vi "main.vi"() -> ()   [LabVIEW 2020]
uses:
  Monochromator/Monochromator.lvclass
  MonoStateFactory/MonoStateFactory.lvclass
  ts_labview_tcp/TCPServer/TCPServer.lvclass
  C:/Users/ecoughlin/repos/ss_monochromator_2/ts_labview_tcp/TCPCommunicator/TCPCommunicator.lvclass
  ts_labview_tcp/TCPComEvents/TCPComEvents.lvclass
  MonoCommunicator/MonoCommunicator.lvclass
  MonoPubSubData/MonoPubSubData.lvclass
  Typedefs/SWStatus.ctl
  ts_labview_tcp/TCPSettings/TCPSettings.lvclass
  MonoPubSubData/MonoPubSubData.lvclass/MonoPubSubData.ctl
  ts_labview_tcp/TCPComEvents/TCPComEvents.lvclass/TCPComEvents.ctl
  ts_labview_tcp/TCPCommunicator/TCPCommunicator.lvclass/TCPCommunicator.ctl
  MonoCommunicator/MonoCommunicator.lvclass/MonoCommunicator.ctl
  Monochromator/Monochromator.lvclass/Monochromator.ctl
  MonoSettings/Settings/ProcessSetting/ProcessSettings.lvclass
  C:/Users/ecoughlin/repos/ss_monochromator_2/WindowsController/MonoSettings/Settings/Settings/Setting.lvclass
  MonoSettings/Settings/Settings/Setting.lvclass/Setting.ctl
  ts_labview_tcp/TCPCommunicator/TCPCommunicator.lvclass
  MonoSettings/Settings/Settings/Setting.lvclass
  MonoSettings/Settings/ConfigurationFileReader/ConfigurationFileReader.lvclass
panel:
  out "TCP Connected":bool
  out "MonoID":string(combo)="Mono4"
  out "UniqueID":string="Mono1"
  # "Monochrmator"
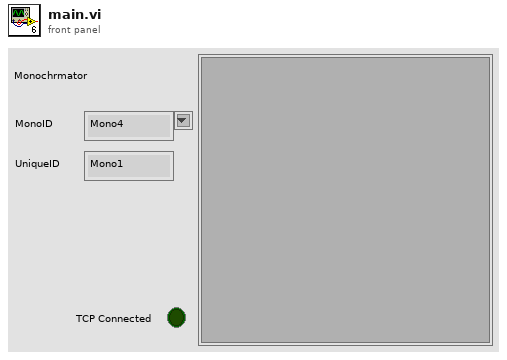
[diagram p1: front panel]
types:
  T1 = typedef "SWStatus.ctl" = enum16{"OfflineState", "ReadyState", "SettingUpState", "FaultState"}
  T2 = typedef "Settings.lvlib/ConfigurationTypedefs.lvlib/MonochromatorSettings.ctl" = cluster{"Force Init":bool, "WavelengthMin":T3, "WavelengthMax":T3, "SlitWidthMin":T4, "SlitWidthMax":T4, "timeout":dbl}
  T3 = typedef "wavelength.ctl" = dbl
  T4 = typedef "slitWidth.ctl" = dbl
  T5 = typedef "Settings.lvlib/ConfigurationTypedefs.lvlib/TCPConfiguration.ctl" = cluster{"IP":string, "port_low":u16, "port_up":u16, "connection_timeout ":i32, "reading_timeout":i32, "writing_timeout":i32}
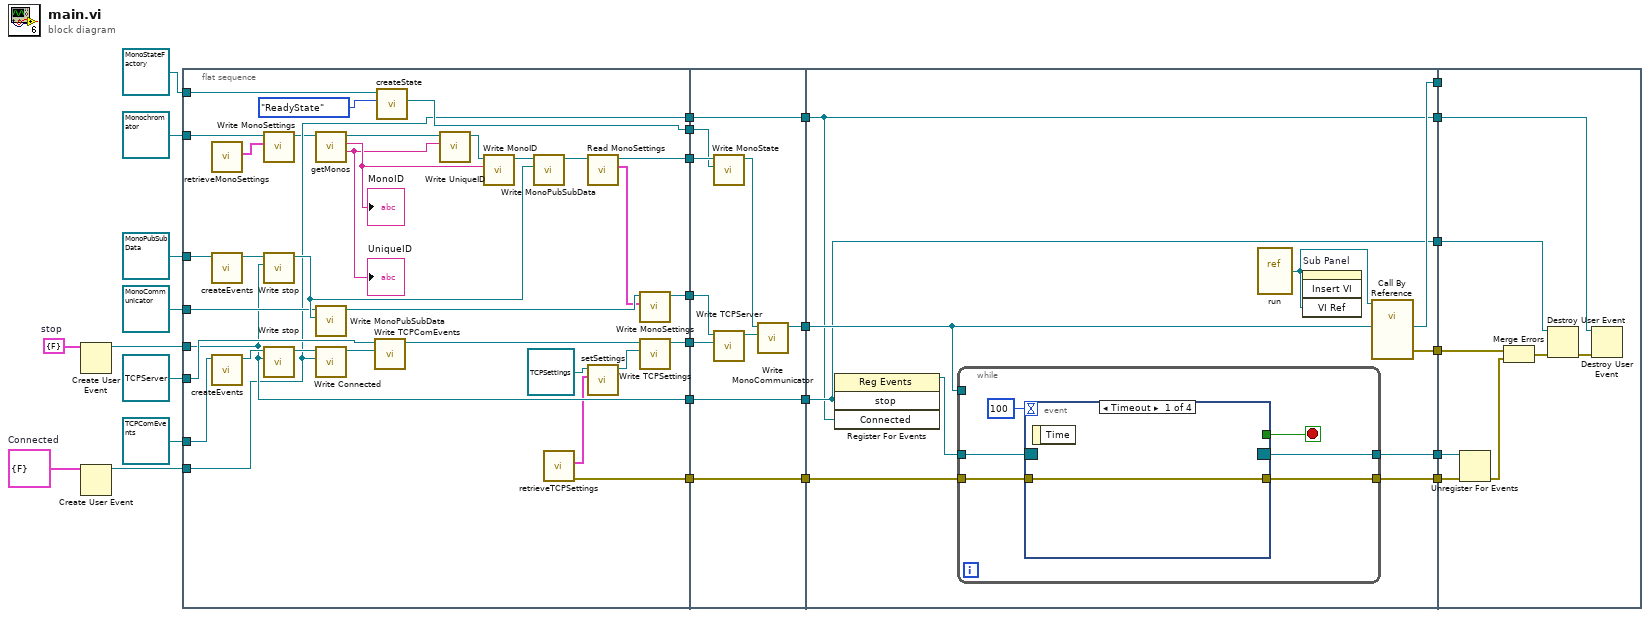
[diagram p0: block diagram]
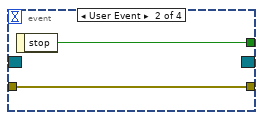
[diagram p2: hidden frame]
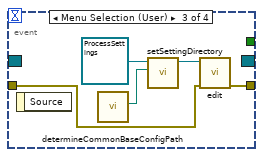
[diagram p3: hidden frame]
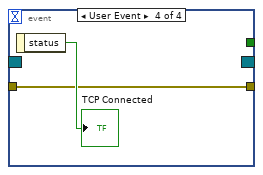
[diagram p4: hidden frame]
diagram:
  w6 = cluster{"status":bool} {"status"=FALSE}  # Connected
  w21 = cluster{"stop":bool} {"stop"=FALSE}  # stop
  n1 = Create User Event(user event datatype=w21) -> (user event=w20:refnum<user-event>)  [unwired: 1 in, 1 out]
  n2 = Create User Event(user event datatype=w6) -> (user event=w5:refnum<user-event>)  [unwired: 1 in, 1 out]
  n3 = flat-sequence {
    tunnel: [w29] -> w26
    tunnel: [w58] -> w24
    tunnel: [w53] -> w19
    tunnel: [w31] -> w16
    tunnel: [w48] -> w12
    tunnel: refnum<class "Monochromator.lvclass"> refnum ("Monochromator.lvclass") -> [w37]
    tunnel: refnum<class "MonoStateFactory.lvclass"> refnum ("MonoStateFactory.lvclass") -> [w60]
    tunnel: refnum<class "TCPComEvents.lvclass"> refnum ("TCPComEvents.lvclass") -> [w57]
    tunnel: refnum<class "TCPServer.lvclass"> refnum ("TCPServer.lvclass") -> [w55]
    tunnel: w20 -> [w48]
    tunnel: refnum<class "MonoPubSubData.lvclass"> refnum ("MonoPubSubData.lvclass") -> [w52]
    tunnel: refnum<class "MonoCommunicator.lvclass"> refnum ("MonoCommunicator.lvclass") -> [w49]
    tunnel: [w35] -> w8
    tunnel: w5 -> [w39]
    tunnel: [w39] -> w3
    tunnel: w26 -> [w70]
    tunnel: w24 -> [w69]
    tunnel: w19 -> [w67]
    tunnel: w16 -> [w68]
    tunnel: [w64] -> w15
    tunnel: [w63] -> w13
    tunnel: w12 -> [w63]
    tunnel: [w62] -> w9
    tunnel: w8 -> [w62]
    tunnel: [w61] -> w4
    tunnel: w3 -> [w61]
    tunnel: w15 -> [w77]
    tunnel: [w76] -> w14
    tunnel: w13 -> [w76]
    tunnel: [w79] -> w11
    tunnel: [w78] -> w10
    tunnel: w9 -> [w74]
    tunnel: [w73] -> w7
    tunnel: w4 -> [w71]
    tunnel: [w72] -> w2
    tunnel: [w71] -> w1
    tunnel: w14 -> [w104]
    tunnel: w11 -> [_]
    tunnel: w10 -> [w103]
    tunnel: w7 -> [w98]
    tunnel: w2 -> [w99]
    tunnel: w1 -> [w100]
    frame #0 {
      n4 = call "retrieveMonoSettings.vi"() -> ("Mono Settings"=w36:T2)  [unwired: 9 in, 2 out]
      n5 = call "createEvents.vi"("MonoPubSubData in"=w52) -> ("MonoPubSubData out"=w51:refnum<class "MonoPubSubData.lvclass">)  [unwired: 9 in, 1 out]
      n6 = call "createEvents.vi"("TCPComEvents in"=w57) -> ("TCPComEvents out"=w56:refnum<class "TCPComEvents.lvclass">)  [unwired: 9 in, 1 out]
      n7 = call "Write MonoSettings.vi"("SetLimits"=w36, "Monochromator in"=w37) -> ("Monochromator out"=w38:refnum<class "Monochromator.lvclass">)  [unwired: 8 in, 1 out]
      n8 = call "Write stop.vi"("stop"=w48, "MonoPubSubData in"=w51) -> ("MonoPubSubData out"=w50:refnum<class "MonoPubSubData.lvclass">)  [unwired: 8 in, 1 out]
      n9 = call "Write stop.vi"("stop"=w48, "TCPComEvents in"=w56) -> ("TCPComEvents out"=w41:refnum<class "TCPComEvents.lvclass">)  [unwired: 8 in, 1 out]
      n10 = call "getMonos.vi"("Monochromator in"=w38) -> ("Current UniqueID"=w43:string, "Mono ID"=w44:string, "Monochromator out"=w45:refnum<class "Monochromator.lvclass">)  [unwired: 6 in, 2 out]
      "UniqueID" <- w43
      "MonoID" <- w44
      n11 = call "Write MonoPubSubData.vi"("MonoPubSubData.lvclass"=w50, "MonoCommunicator in"=w49) -> ("MonoCommunicator out"=w33:refnum<class "MonoCommunicator.lvclass">)  [unwired: 8 in, 1 out]
      n12 = call "Write Connected.vi"("Connected"=w39, "TCPComEvents in"=w41) -> ("TCPComEvents out"=w40:refnum<class "TCPComEvents.lvclass">)  [unwired: 8 in, 1 out]
      n13 = call "Write TCPComEvents.vi"("TCPComEvents.lvclass"=w40, "TCPCommunicator in"=w55) -> ("TCPCommunicator out"=w54:refnum<class "TCPServer.lvclass">)  [unwired: 8 in, 1 out]
      n14 = call "createState.vi"("SWStatus"=SWStatus."ReadyState", "MonoStateFactory in"=w60) -> ("MonoState.lvclass"=w58:refnum<class "MonoState.lvclass">)  [unwired: 7 in, 2 out]
      n15 = call "Write UniqueID.vi"("UniqueID"=w43, "Monochromator in"=w45) -> ("Monochromator out"=w47:refnum<class "Monochromator.lvclass">)  [unwired: 8 in, 1 out]
      n16 = call "Write MonoID.vi"("MonoID"=w44, "Monochromator in"=w47) -> ("Monochromator out"=w46:refnum<class "Monochromator.lvclass">)  [unwired: 8 in, 1 out]
      n17 = call "Write MonoPubSubData.vi"("MonoPubSubData.lvclass"=w50, "Monochromator in"=w46) -> ("Monochromator out"=w30:refnum<class "Monochromator.lvclass">)  [unwired: 8 in, 1 out]
      n18 = call "retrieveTCPSettings.vi"() -> ("error out"=w35:errorcluster, "TCPConfiguration"=w32:T5)  [unwired: 9 in, 1 out]
      n19 = call "Read MonoSettings.vi"("Monochromator in"=w30) -> ("Settings"=w28:T2, "Monochromator out"=w29:refnum<class "Monochromator.lvclass">)  [unwired: 8 in, 1 out]
      n20 = call "setSettings.vi"("Settings"=w32, "TCPSettings in"=refnum<class "TCPSettings.lvclass"> refnum) -> ("TCPSettings out"=w42:refnum<class "TCPSettings.lvclass">)  [unwired: 8 in, 1 out]
      n21 = call "Write MonoSettings.vi"("MonoSettings"=w28, "MonoCommunicator in"=w33) -> ("MonoCommunicator out"=w31:refnum<class "MonoCommunicator.lvclass">)  [unwired: 8 in, 1 out]
      n22 = call-dynamic "Write TCPSettings.vi"("TCPSettings.lvclass"=w42, "TCPCommunicator in"=w54) -> ("TCPCommunicator out"=w53:refnum<class "TCPServer.lvclass">)  [unwired: 8 in, 1 out]
    }
    frame #1 {
      n23 = call "Write MonoState.vi"("MonoState.lvclass"=w69, "Monochromator in"=w70) -> ("Monochromator out"=w66:refnum<class "Monochromator.lvclass">)  [unwired: 8 in, 1 out]
      n24 = call "Write TCPServer.vi"("TCPServer.lvclass"=w67, "MonoCommunicator in"=w68) -> ("MonoCommunicator out"=w65:refnum<class "MonoCommunicator.lvclass">)  [unwired: 8 in, 1 out]
      n25 = call "Write MonoCommunicator.vi"("MonoCommunicator.lvclass"=w65, "Monochromator in"=w66) -> ("Monochromator out"=w64:refnum<class "Monochromator.lvclass">)  [unwired: 8 in, 1 out]
    }
    frame #2 {
      n26 = register-events(w76, w71) -> (reference out=w75:refnum<event-registration>)  [unwired: 2 in, 1 out]
      n27 = while {
        tunnel: w77 -> [_]
        tunnel: w75 -> [w86]
        tunnel: w74 -> [w83]
        tunnel: [w82] -> w73
        tunnel: [w81] -> w72
        stop <- w85 stop-if-true
        n28 = event shown="[0] Timeout" {
          selector: w86 -> [_ _ _ _]
          dyn-events: [_ _ _ _] -> w81
          timeout: 100 -> [_ _ _ _]
          tunnel: [_ w89 _ _] -> w85
          tunnel: w83 -> [w87 w88 w93 w95]
          tunnel: [w87 w88 w91 w95] -> w82
          event Timeout {
            n29 = event-data() -> ()  [unwired: 1 in, 1 out]
          }
          event User Event {
            n30 = event-data() -> ("stop"=w89:bool)  [unwired: 1 in]
          }
          event Menu Selection (User) {
            n31 = event-data() -> ()  [unwired: 1 in, 1 out]
            n32 = call "determineCommonBaseConfigPath.vi"() -> ("ConfigurationPath"=w94:path)  [unwired: 9 in, 2 out]
            n33 = call "setSettingDirectory.vi"("SettingDirectory"=w94, "BaseSetting in"=refnum<class "ProcessSettings.lvclass"> refnum ("Settings.lvlib:ProcessSettings.lvclass")) -> ("BaseSetting out"=w92:refnum<class "ProcessSettings.lvclass">)  [unwired: 9 in]
            n34 = call-dynamic "edit.vi"("error in (no error)"=w93, "BaseSetting in"=w92) -> ("error out"=w91:errorcluster)  [unwired: 7 in, 2 out]
          }
          event User Event {
            n35 = event-data() -> ("status"=→"TCP Connected":bool)  [unwired: 1 in]
          }
        }
      }
      n36 = vi-ref "run.vi"() -> (w80:refnum<vi>)
      n37 = invoke on="Sub Panel" class="SubPnl" method="Insert VI"("VI Ref"=w80) -> ()  [unwired: 3 in, 4 out]
      n38 = call-by-ref "?"(reference=w80, "Monochromator in"=w77) -> ("error out"=w78:errorcluster, "Monochromator out"=w79:refnum<class "Monochromator.lvclass">)  [unwired: 10 in, 2 out]
    }
    frame #3 {
      n39 = Unregister For Events(event registration refnum=w99, error in=w98) -> (error out=w97:errorcluster)
      n40 = Merge Errors(w103, w97) -> (w102:errorcluster)
      n41 = Destroy User Event(user event=w104, error in=w102) -> (error out=w101:errorcluster)
      n42 = Destroy User Event(user event=w100, error in=w101) -> ()  [unwired: 1 out]
    }
  }
